vi "PID sensor no reset.vi"(4 "State":i16, 5 "Time":dbl format="%.2f", 6 "Sensor Values":dbl[](array[numeric]), 7 "Set Points":dbl[](array[numeric])) -> (0 "required data":T1={"Set Point names"=["target value", "P Kc", "I Ti (s)", "D Td (s)"], "required number of setpoints"=4, "required number of sensors"=1, "Sensor names"=["Measured process value"]}, 3 "output value":dbl)   [LabVIEW 2019]
uses:
  <vilib>/addons/control/pid/pid.llb/PID (DBL).vi
  <vilib>/addons/control/pid/NI_PID_pid.lvlib
panel:
  # "Enter the correct information for this control code in the required data structure below. Then make the current value default by right clicking on the border of the data structure."
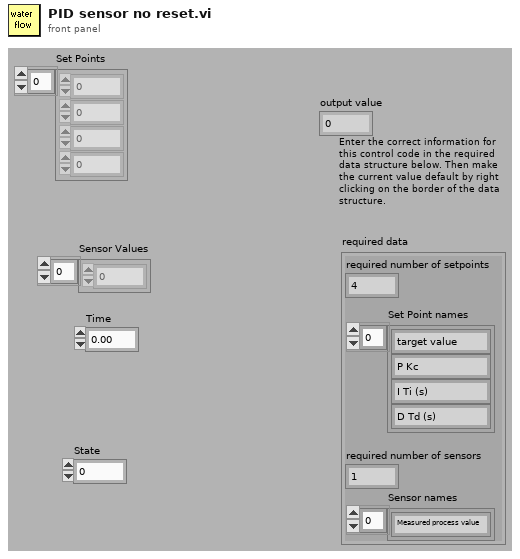
[diagram p1: front panel]
types:
  T1 = cluster{"Set Point names":string[], "required number of setpoints":u8, "required number of sensors":u8, "Sensor names":string[]}
  T2 = cluster{"Set Points[0]":dbl, "Set Points[1]":dbl, "Set Points[2]":dbl, "Set Points[3]":dbl}
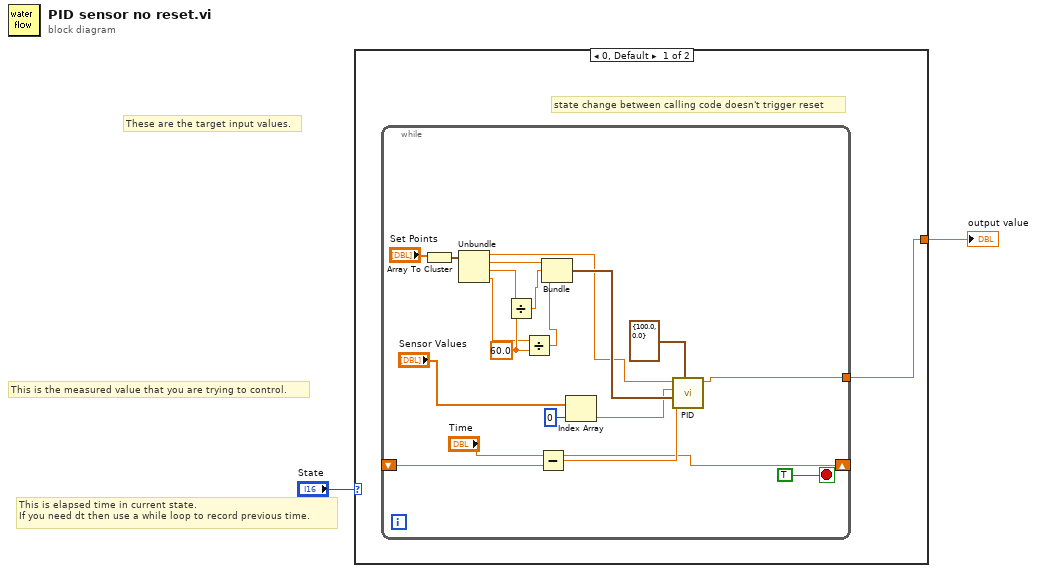
[diagram p0: block diagram]
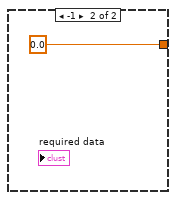
[diagram p2: hidden frame]
diagram:
  # "These are the target input values."
  # "This is the measured value that you are trying to control."
  # "This is elapsed time in current state.\nIf you need dt then use a while loop to record previous time."
  n1 = case shown="0, Default" "State" {
    tunnel: [w3 0.0 ("fraction on")] -> w2
    frame 0, Default {
      # "state change between calling code doesn't trigger reset"
      n2 = while {
        shift-right: ["Time"] -> _
        shift-left: _ -> [w21]
        tunnel: [w9] -> w3
        stop <- TRUE stop-if-true
        w8 = 60.0 ("y")
        n3 = Array To Cluster(array="Set Points") -> (cluster=w16:T2)
        n4 = Unbundle(w16) -> ("Set Points[0]"=w10:dbl, "Set Points[1]"=w15:dbl, "Set Points[2]"=w6:dbl, "Set Points[3]"=w7:dbl)
        n5 = Divide(x=w6, y=w8) -> (x/y=w5:dbl)
        n6 = Divide(x=w7, y=w8) -> (x/y=w4:dbl)
        n7 = Subtract(x="Time", y=w21) -> (x-y=w20:dbl)
        n8 = Bundle("Set Points[1]"=w15, w5, w4) -> (w14:cluster{"Set Points[1]":dbl, dbl, dbl})  [unwired: 1 in]
        n9 = Index Array(array="Sensor Values", index=0) -> (element=w11:dbl)
        n10 = call-poly <vilib>:"PID.vi"("output range"=cluster{"output high":dbl, "output low":dbl} {"output high"=100.0, "output low"=0.0}, "dt (s)"=w20, "PID gains"=w14, "process variable"=w11, "setpoint"=w10) -> ("output"=w9:dbl)  [unwired: 5 in, 1 out]
      }
    }
    frame -1 {
    }
  }
  "output value" <- w2
